vi "Set Memory.vi"(0 "connection ID":refnum<k16>, 1 "address":u32, 2 "port":u16, 5 "Digital Number":u16, 7 "Data":i16, 9 "timeout ms (1000)":i32=1000, 11 "error in (no error)":errorcluster) -> (4 "connection ID out":refnum<k16>, 6 "received data":string, 15 "error out":errorcluster)   [LabVIEW 2016, in "instr.lvlib"]
doc: "Sets given memory item to given value."
uses:
  instr.lvlib
panel:
  out "Send String":string
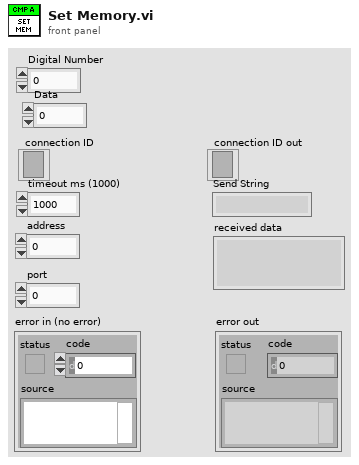
[diagram p1: front panel]
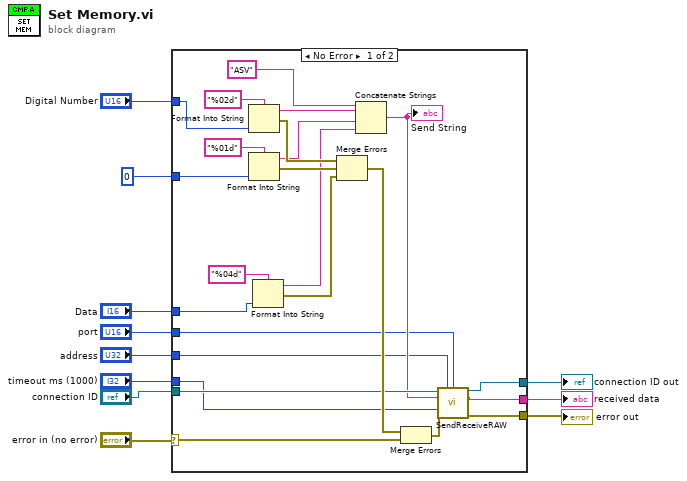
[diagram p0: block diagram]
diagram:
  n1 = case shown="No Error" "error in (no error)" {
    selector: "error in (no error)" -> [w30 w37]
    tunnel: [w26 w37] -> w11
    tunnel: [w25 _] -> w9
    tunnel: "timeout ms (1000)" -> [w21 _]
    tunnel: "connection ID" -> [w23 w36]
    tunnel: [w24 w36] -> w6
    tunnel: "Digital Number" -> [w16 _]
    tunnel: "address" -> [w19 _]
    tunnel: "port" -> [w18 _]
    tunnel: "Data" -> [w15 _]
    tunnel: i16 0 ("Data 2") -> [w13 _]
    frame No Error {
      n2 = Format Into String(format string="%02d", w16) -> (resulting string=w28:string, error out=w32:errorcluster)  [unwired: 2 in]
      n3 = Format Into String(format string="%01d", w13) -> (resulting string=w27:string, error out=w31:errorcluster)  [unwired: 2 in]
      n4 = Format Into String(format string="%04d", w15) -> (resulting string=w12:string, error out=w14:errorcluster)  [unwired: 2 in]
      n5 = Merge Errors(w32, w31, w14) -> (w29:errorcluster)
      n6 = Concatenate Strings("ASV" ("data in"), w28, w27, w12) -> (w20:string)
      "Send String" <- w20
      n7 = Merge Errors(w29, w30) -> (w22:errorcluster)
      n8 = call "SendReceiveRAW.vi"("connection ID"=w23, "address"=w19, "port"=w18, "RAW data in"=w20, "timeout ms (1000)"=w21, "error in (no error)"=w22) -> ("connection ID out"=w24:refnum<k16>, "received data"=w25:string, "error out"=w26:errorcluster)  [unwired: 7 in]
    }
    frame Error {
    }
  }
  "error out" <- w11
  "received data" <- w9
  "connection ID out" <- w6
